vi "Convert Mouse POS to Lat Long.vi"(8 "Error In":errorcluster, 10 "GMap Position":T1, 11 "Mouse Position":T1) -> (0 "Error Out":errorcluster, 1 "Lng":dbl, 2 "Lat":dbl, 3 "Point Ref":refnum<k24>)   [LabVIEW 2014]
uses:
  <vilib>/Utility/miscctls.llb/LVPositionTypeDef.ctl
  C:/Robotic Systems/Products/AgFalcon/Software/Ground Station/Data/Mapping DLL/GMap.NET.Core.dll
  Data/Mapping DLL/GMap.NET.Core.dll
  C:/Robotic Systems/Products/AgFalcon/Software/Ground Station/Data/Mapping DLL/GMap.NET.WindowsForms.dll
  Data/Mapping DLL/GMap.NET.WindowsForms.dll
  Reference/SubVI/GMap DLL Refernce.vi
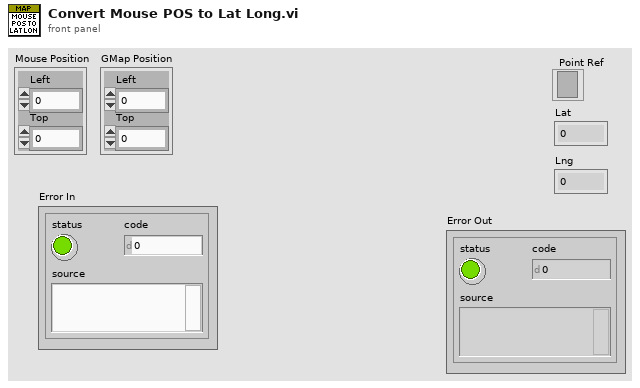
[diagram p1: front panel]
types:
  T1 = typedef "LVPositionTypeDef.ctl" = cluster{"Left":i32, "Top":i32}
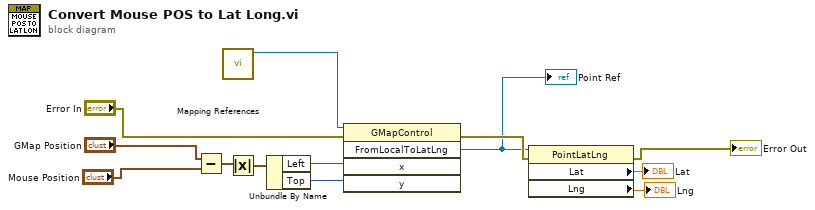
[diagram p0: block diagram]
diagram:
  n1 = Subtract(x="GMap Position", y="Mouse Position") -> (x-y=w4:T1)
  n2 = call-poly "Mapping References.vi"() -> ("GMap DLL Reference"=w5:refnum<k24>)  [unwired: 10 in, 1 out]
  n3 = Absolute Value(x=w4) -> (abs(x)=w11:T1)
  n4 = Unbundle By Name(w11) -> ("Left"=w10:i32, "Top"=w9:i32)
  n5 = invoke class="GMapControl" method="FromLocalToLatLng"(reference=w5, error in="Error In", "x"=w10, "y"=w9) -> (error out=w7:errorcluster, "FromLocalToLatLng"=w1:refnum<k24>)  [unwired: 1 in, 3 out]
  "Point Ref" <- w1
  n6 = property class="PointLatLng"(reference=w1, error in=w7) -> (error out=→"Error Out":errorcluster, "Lat"=→"Lat":dbl, "Lng"=→"Lng":dbl)  [unwired: 1 out]
